vi "MaxHeight.vi"(0 "Extension Length":dbl, 1 "Pivot Angle":dbl, 3 "Wrist Angle (relative to ground)":dbl, 4 "Claw Angle":dbl=1.57) -> (13 "Max Extension":dbl, 14 "Disable Extend":bool, 15 "Disable Pivot Forward":bool, 16 "Disable Pivot Back":bool, 17 "Disable Wrist Forward":bool, 18 "Disable Wrist Back":bool, 19 "Disable Claw Close":bool)   [LabVIEW 2014]
uses:
  Robot Global Data.vi
panel:
  out "Wrist Above Max Height":bool
  out "Claw Above Max Height":bool
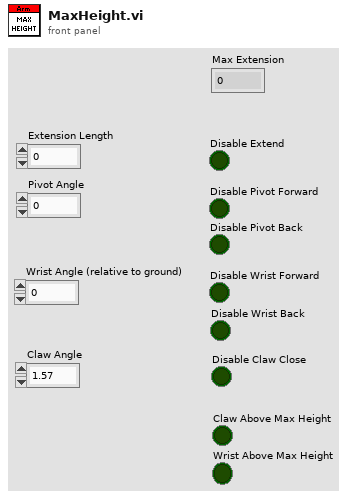
[diagram p1: front panel]
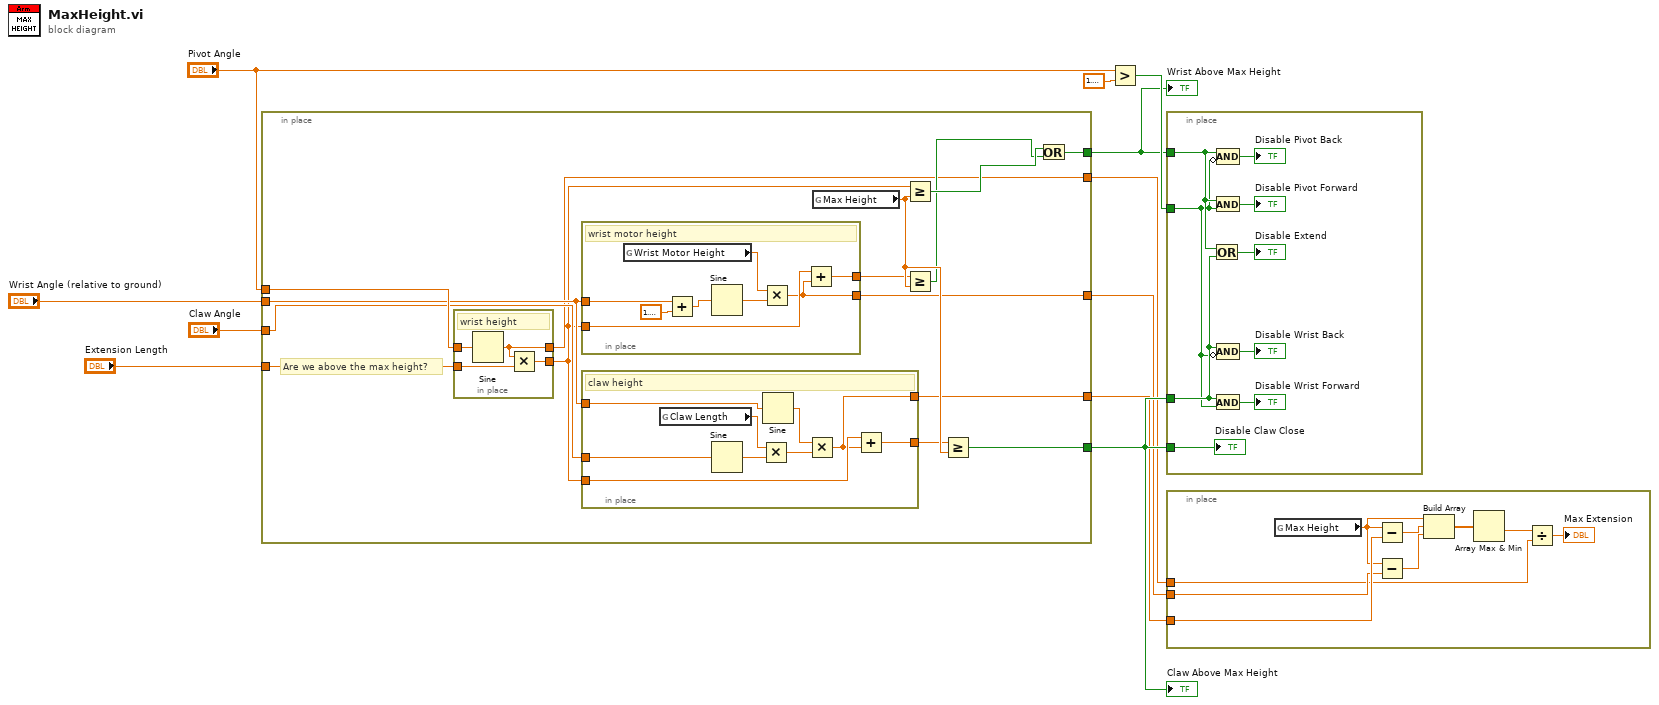
[diagram p0: block diagram]
diagram:
  n1 = in-place {
    in-place-border: [w18] -> w5
    in-place-border: "Extension Length" -> [w26]
    in-place-border: "Wrist Angle (relative to ground)" -> [w21]
    in-place-border: "Pivot Angle" -> [w25]
    in-place-border: [w24] -> w4
    in-place-border: "Claw Angle" -> [w23]
    in-place-border: [w14] -> w3
    in-place-border: [w13] -> w2
    in-place-border: [w12] -> w1
    # "Are we above the max height?"
    n2 = in-place {
      in-place-border: w26 -> [w30]
      in-place-border: w25 -> [w29]
      in-place-border: [w28] -> w16
      in-place-border: [w27] -> w12
      # "wrist height"
      n3 = Sine(x=w29) -> (sin(x)=w27:dbl)
      n4 = Multiply(x=w27, y=w30) -> (x*y=w28:dbl)
    }
    n5 = in-place {
      in-place-border: [w42] -> w15
      in-place-border: w21 -> [w44]
      in-place-border: w16 -> [w41]
      in-place-border: [w40] -> w13
      # "wrist motor height"
      n6 = global read "Robot Global Data.vi" "Wrist Motor Height"() -> (w43:dbl)
      n7 = Add(x=w44, y=1.5707963267948966) -> (x+y=w46:dbl)
      n8 = Sine(x=w46) -> (sin(x)=w47:dbl)
      n9 = Multiply(x=w43, y=w47) -> (x*y=w40:dbl)
      n10 = Add(x=w41, y=w40) -> (x+y=w42:dbl)
    }
    n11 = in-place {
      in-place-border: [w33] -> w17
      in-place-border: w23 -> [w36]
      in-place-border: w21 -> [w34]
      in-place-border: w16 -> [w32]
      in-place-border: [w31] -> w14
      # "claw height"
      n12 = global read "Robot Global Data.vi" "Claw Length"() -> (w35:dbl)
      n13 = Sine(x=w36) -> (sin(x)=w37:dbl)
      n14 = Multiply(x=w35, y=w37) -> (x*y=w38:dbl)
      n15 = Sine(x=w34) -> (sin(x)=w39:dbl)
      n16 = Multiply(x=w39, y=w38) -> (x*y=w31:dbl)
      n17 = Add(x=w32, y=w31) -> (x+y=w33:dbl)
    }
    n18 = global read "Robot Global Data.vi" "Max Height"() -> (w20:dbl)
    n19 = Greater Or Equal?(x=w16, y=w20) -> (x >= y?=w22:bool)
    n20 = Greater Or Equal?(x=w15, y=w20) -> (x >= y?=w19:bool)
    n21 = Greater Or Equal?(x=w17, y=w20) -> (x >= y?=w24:bool)
    n22 = Or(x=w22, y=w19) -> (x .or. y?=w18:bool)
  }
  "Claw Above Max Height" <- w4
  "Wrist Above Max Height" <- w5
  n23 = Greater?(x="Pivot Angle", y=1.5707963267948966) -> (0:w6:bool)
  n24 = in-place {
    in-place-border: w5 -> [w54]
    in-place-border: w4 -> [w51]
    in-place-border: w6 -> [w50]
    in-place-border: w4 -> [w48]
    n25 = Or(x=w54, y=w51) -> (x .or. y?=→"Disable Extend":bool)
    n26 = And(x=w54, y=w50) -> (x .and. y?=→"Disable Pivot Forward":bool)
    n27 = And(x=w51, y=w50) -> (x .and. y?=→"Disable Wrist Forward":bool)
    n28 = Compound Arithmetic op=AND(w54, invert w50) -> (→"Disable Pivot Back":bool)
    n29 = Compound Arithmetic op=AND(w51, invert w50) -> (→"Disable Wrist Back":bool)
    "Disable Claw Close" <- w48
  }
  n30 = in-place {
    in-place-border: w3 -> [w64]
    in-place-border: w2 -> [w61]
    in-place-border: w1 -> [w58]
    n31 = global read "Robot Global Data.vi" "Max Height"() -> (w62:dbl)
    n32 = Subtract(x=w62, y=w64) -> (x-y=w65:dbl)
    n33 = Subtract(x=w62, y=w61) -> (x-y=w63:dbl)
    n34 = Build Array(w62, w65, w63) -> (w60:dbl[])
    n35 = Array Max & Min(array=w60) -> (min value=w59:dbl)  [unwired: 3 out]
    n36 = Divide(x=w59, y=w58) -> (x/y=→"Max Extension":dbl)
  }
